vi "Init Control Indices Map.vi"(8 "error in":errorcluster, 10 "VI Refnum":refnum<vi>, 11 "Panel Actor Template in":refnum<class "Network Management UI.lvclass">) -> (0 "error out":errorcluster, 3 "Panel Actor Template out":refnum<class "Network Management UI.lvclass">)   [LabVIEW 2024, in "Network Management UI.lvlib" / "Network Management UI.lvclass"]
uses:
  Network Management UI.lvclass
  Network Management UI.lvclass/Network Management UI.ctl
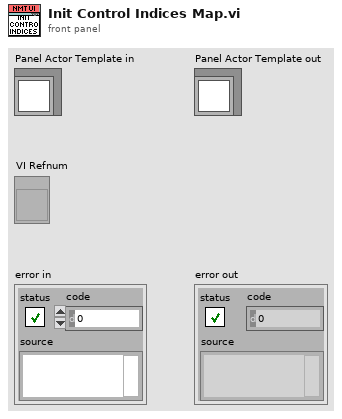
[diagram p1: front panel]
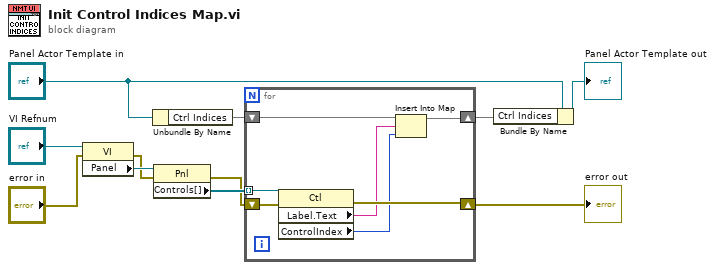
[diagram p0: block diagram]
diagram:
  n1 = property class="VI"(reference="VI Refnum", error in="error in") -> (error out=w9:errorcluster, "Panel"=w10:refnum<vi>)  [unwired: 1 out]
  n2 = Unbundle By Name("Panel Actor Template in") -> ("Ctrl Indices"=w6:map{string, i32})
  n3 = property class="Pnl"(reference=w10, error in=w9) -> (error out=w7:errorcluster, "Controls[]"=w8:refnum<vi>[])  [unwired: 1 out]
  n4 = for {
    tunnel: w8 -> [w18] mode=indexing
    shift-right: [w16] -> w1
    shift-left: w7 -> [w17]
    shift-right: [w14] -> w5
    shift-left: w6 -> [w15]
    n5 = property class="Ctl"(reference=w18, error in=w17) -> (error out=w16:errorcluster, "Label.Text"=w13:string, "ControlIndex"=w12:i32)  [unwired: 1 out]
    n6 = Insert Into Map(map in=w15, key=w13, value=w12) -> (map out=w14:map{string, i32})  [unwired: 2 out]
  }
  "error out" <- w1
  n7 = Bundle By Name(cluster="Panel Actor Template in", "Ctrl Indices"=w5) -> (→"Panel Actor Template out":refnum<class "Network Management UI.lvclass">)
